vi "Get Error.vi"(11 "Actor in":refnum<class "Actor.lvclass">) -> (2 "Error":errorcluster)   [LabVIEW 2021, in "Actor.lvclass"]
uses:
  Actor.lvclass
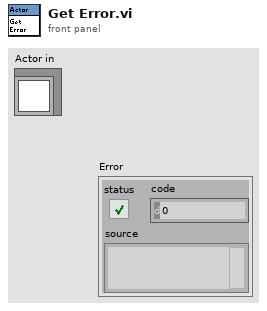
[diagram p1: front panel]
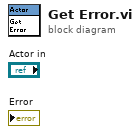
[diagram p0: block diagram]
diagram:
